vi "Process Ack Data - Open SVs.vi"(8 "error in (no error)":errorcluster, 9 "CPU Load Data":variant, 11 "SV B-M (Host) in":refnum<class "SV B-M (Host).lvclass">) -> (0 "error out":errorcluster, 3 "SV B-M (Host) out":refnum<class "SV B-M (Host).lvclass">)   [LabVIEW 2015, in "SV B-M (Host).lvclass"]
uses:
  SV B-M (Host).lvclass
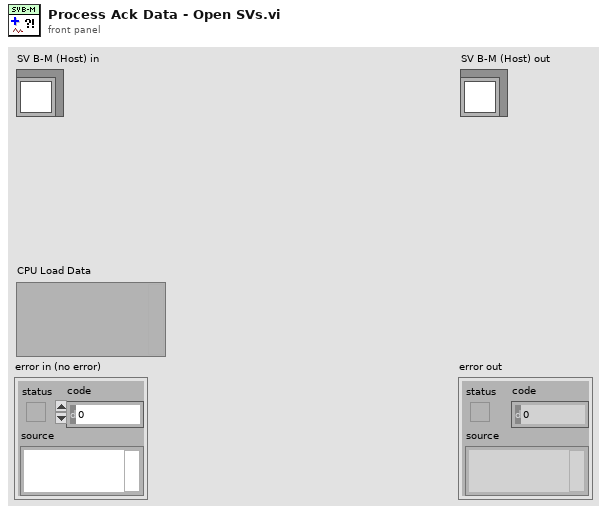
[diagram p1: front panel]
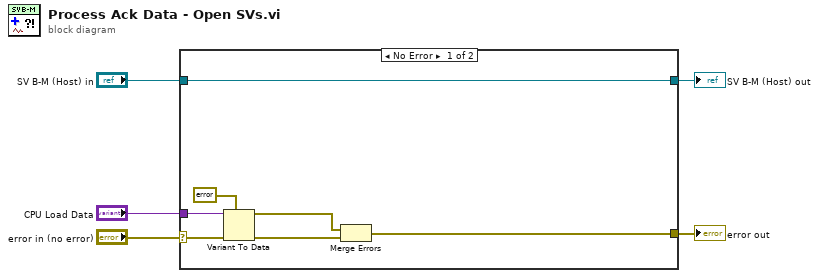
[diagram p0: block diagram]
diagram:
  n1 = case shown="No Error" "error in (no error)" {
    selector: "error in (no error)" -> [w11 w14]
    tunnel: [w9 w14] -> w4
    tunnel: [w6 w13] -> w2
    tunnel: "SV B-M (Host) in" -> [w6 w13]
    tunnel: "CPU Load Data" -> [w12 _]
    frame No Error {
      n2 = Variant To Data(error in=w11, type=errorcluster {"status"=FALSE, "code"=0, "source"=""} ("error constant"), Variant=w12) -> (data=w7:errorcluster, error out=w10:errorcluster)
      n3 = Merge Errors(w7, w10) -> (w9:errorcluster)
    }
    frame Error {
    }
  }
  "error out" <- w4
  "SV B-M (Host) out" <- w2
